vi "MACMoveBotSpeakVIs.vi"() -> ()   [LabVIEW 2014]
panel:
  out "error out bsLib":errorcluster
  out "new path":path
  out "error out example":errorcluster
  out "new path 4":path
  out "new path 3":path
  out "new path 2":path
  out "error out manager":errorcluster
  out "error bs":errorcluster
  out "total error out":errorcluster
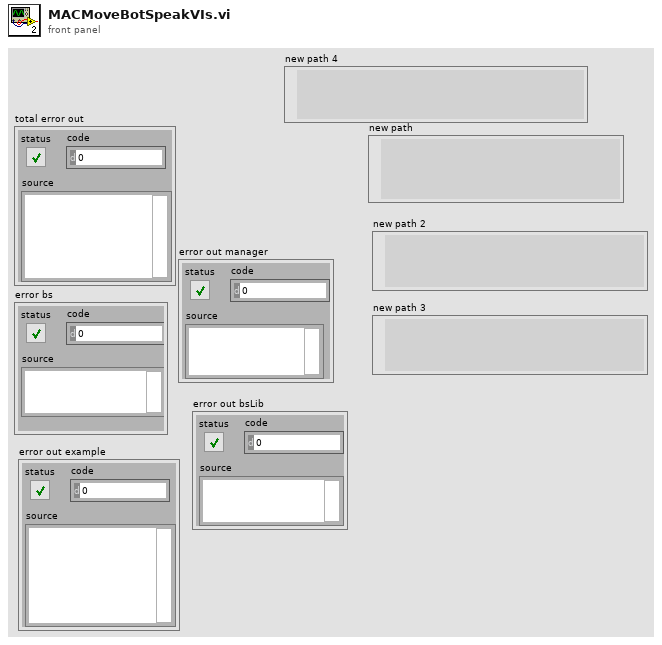
[diagram p1: front panel]
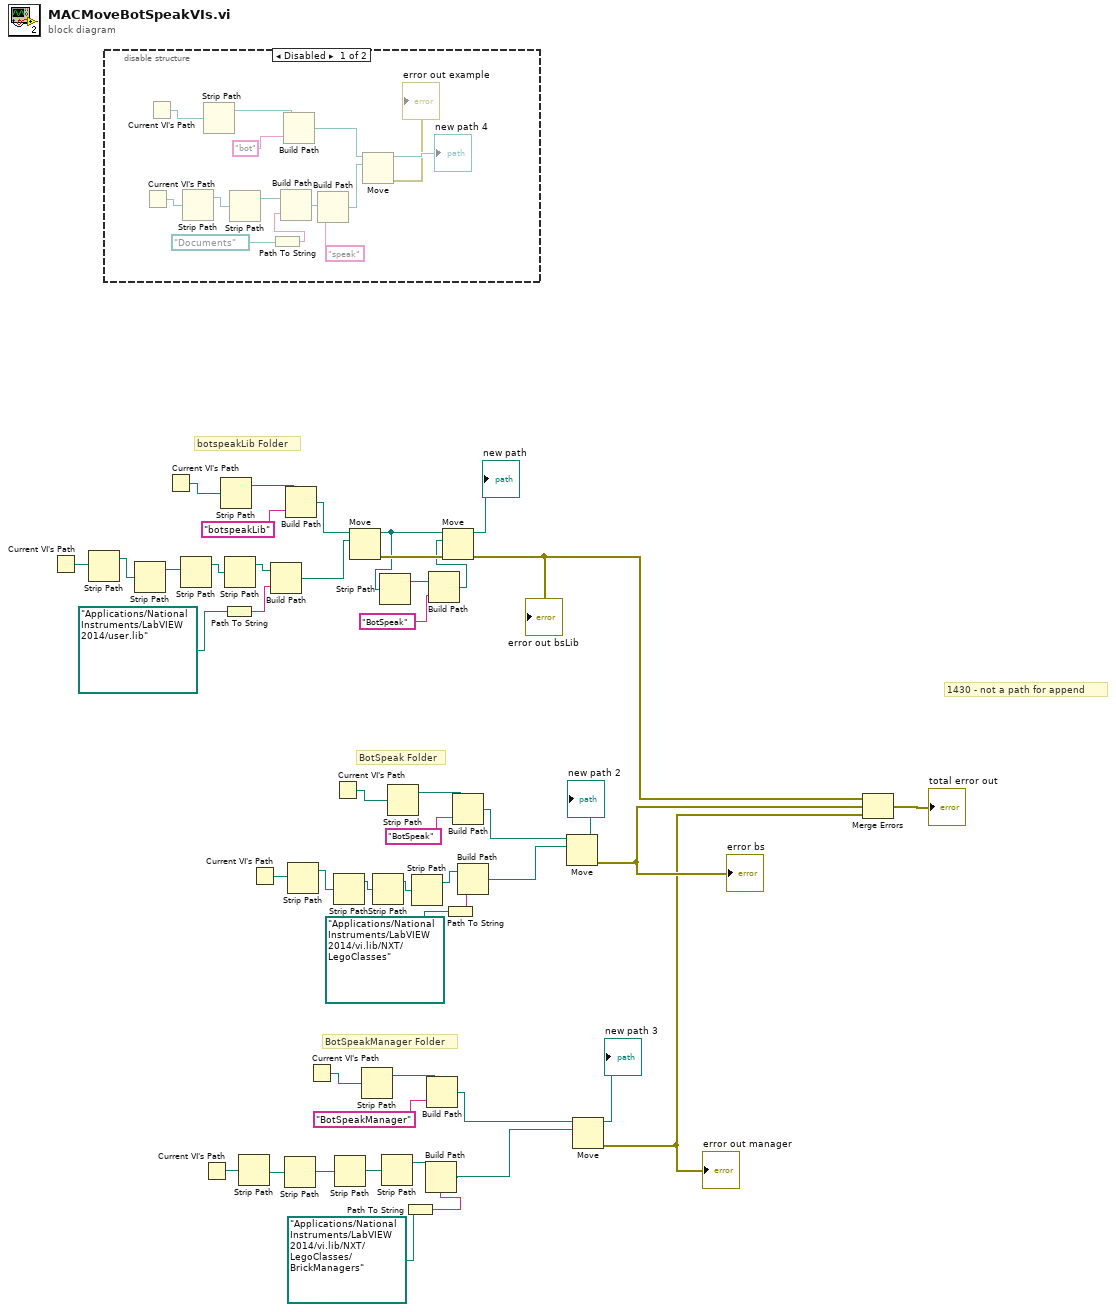
[diagram p0: block diagram]
diagram:
  # "1430 - not a path for append"
  # "BotSpeakManager Folder"
  # "BotSpeak Folder"
  # "botspeakLib Folder"
  n1 = Current VI's Path() -> (path=w44:path)
  n2 = Strip Path(path=w44) -> (stripped path=w43:path)  [unwired: 1 out]
  n3 = disable-structure shown="Disabled" {
    frame Disabled {
      n4 = Current VI's Path() -> (path=w59:path)
      n5 = Current VI's Path() -> (path=w62:path)
      n6 = Strip Path(path=w59) -> (stripped path=w58:path)  [unwired: 1 out]
      n7 = Strip Path(path=w62) -> (stripped path=w61:path)  [unwired: 1 out]
      n8 = Strip Path(path=w58) -> (stripped path=w57:path)  [unwired: 1 out]
      n9 = Path To String(path=path "Documents") -> (string=w51:string)
      n10 = Build Path(base path=w57, name or relative path=w51) -> (appended path=w55:path)
      n11 = Build Path(base path=w61, name or relative path="bot") -> (appended path=w56:path)
      n12 = Build Path(base path=w55, name or relative path="speak") -> (appended path=w54:path)
      n13 = Move(source path=w56, 10:w54) -> (error out=→"error out example":errorcluster, 3:→"new path 4":path)  [unwired: 3 in, 1 out]
    }
    frame Enabled {
    }
  }
  n14 = Strip Path(path=w43) -> (stripped path=w21:path)  [unwired: 1 out]
  n15 = Current VI's Path() -> (path=w48:path)
  n16 = Strip Path(path=w21) -> (stripped path=w20:path)  [unwired: 1 out]
  n17 = Current VI's Path() -> (path=w28:path)
  n18 = Strip Path(path=w48) -> (stripped path=w47:path)  [unwired: 1 out]
  n19 = Path To String(path=path "Applications/National Instruments/LabVIEW 2014/user.lib") -> (string=w41:string)
  n20 = Strip Path(path=w20) -> (stripped path=w19:path)  [unwired: 1 out]
  n21 = Strip Path(path=w28) -> (stripped path=w27:path)  [unwired: 1 out]
  n22 = Current VI's Path() -> (path=w36:path)
  n23 = Build Path(base path=w19, name or relative path=w41) -> (appended path=w8:path)
  n24 = Strip Path(path=w27) -> (stripped path=w15:path)  [unwired: 1 out]
  n25 = Build Path(base path=w47, name or relative path="botspeakLib") -> (appended path=w45:path)
  n26 = Strip Path(path=w36) -> (stripped path=w35:path)  [unwired: 1 out]
  n27 = Current VI's Path() -> (path=w32:path)
  n28 = Current VI's Path() -> (path=w40:path)
  n29 = Strip Path(path=w35) -> (stripped path=w18:path)  [unwired: 1 out]
  n30 = Strip Path(path=w15) -> (stripped path=w14:path)  [unwired: 1 out]
  n31 = Move(source path=w45, 10:w8) -> (error out=w7:errorcluster, 3:w5:path)  [unwired: 3 in, 1 out]
  n32 = Strip Path(path=w32) -> (stripped path=w31:path)  [unwired: 1 out]
  n33 = Strip Path(path=w18) -> (stripped path=w17:path)  [unwired: 1 out]
  n34 = Strip Path(path=w5) -> (stripped path=w4:path)  [unwired: 1 out]
  n35 = Strip Path(path=w14) -> (stripped path=w13:path)  [unwired: 1 out]
  n36 = Strip Path(path=w40) -> (stripped path=w39:path)  [unwired: 1 out]
  n37 = Path To String(path=path "Applications/National Instruments/LabVIEW 2014/vi.lib/NXT/LegoClasses/BrickManagers") -> (string=w26:string)
  n38 = Strip Path(path=w17) -> (stripped path=w16:path)  [unwired: 1 out]
  n39 = Build Path(base path=w13, name or relative path=w26) -> (appended path=w9:path)
  n40 = Build Path(base path=w31, name or relative path="BotSpeakManager") -> (appended path=w29:path)
  n41 = Build Path(base path=w4, name or relative path="BotSpeak") -> (appended path=w2:path)
  n42 = Move(source path=w5, error in=w7, 10:w2) -> (error out=w6:errorcluster, 3:→"new path":path)  [unwired: 2 in, 1 out]
  "error out bsLib" <- w6
  n43 = Path To String(path=path "Applications/National Instruments/LabVIEW 2014/vi.lib/NXT/LegoClasses") -> (string=w33:string)
  n44 = Build Path(base path=w39, name or relative path="BotSpeak") -> (appended path=w37:path)
  n45 = Build Path(base path=w16, name or relative path=w33) -> (appended path=w10:path)
  n46 = Move(source path=w37, 10:w10) -> (error out=w24:errorcluster, 3:→"new path 2":path)  [unwired: 3 in, 1 out]
  "error bs" <- w24
  n47 = Move(source path=w29, 10:w9) -> (error out=w23:errorcluster, 3:→"new path 3":path)  [unwired: 3 in, 1 out]
  "error out manager" <- w23
  n48 = Merge Errors(w6, w24, w23) -> (→"total error out":errorcluster)
